vi "Advantech.vi"(8 "error in (no error)":errorcluster) -> (0 "error out":errorcluster, 3 "Advantech":T1)   [LabVIEW 2012]
panel:
  out "Array":dbl[](array[numeric])
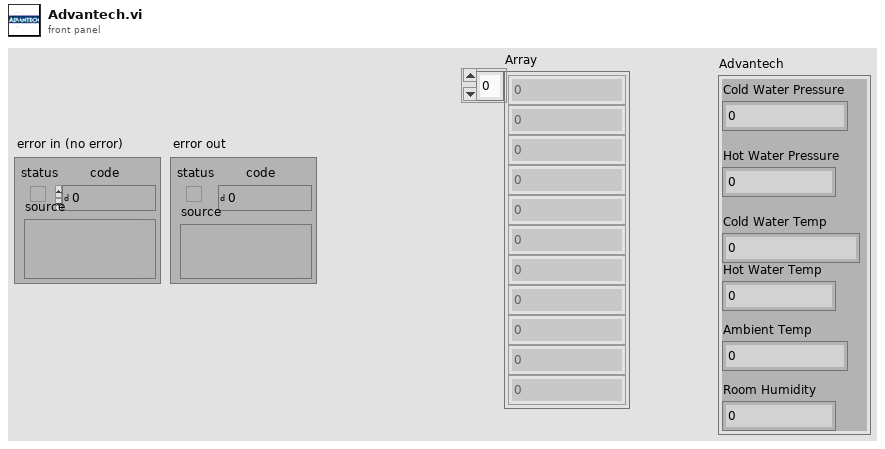
[diagram p1: front panel]
types:
  T1 = cluster{"Cold Water Pressure":dbl, "Hot Water Pressure":dbl, "Cold Water Temp":dbl, "Hot Water Temp":dbl, "Ambient Temp":dbl, "Room Humidity":dbl}
  T2 = cluster{"CP":dbl, "HP":dbl, "F1":dbl, "F2":dbl, "AT":dbl, "RH":dbl}
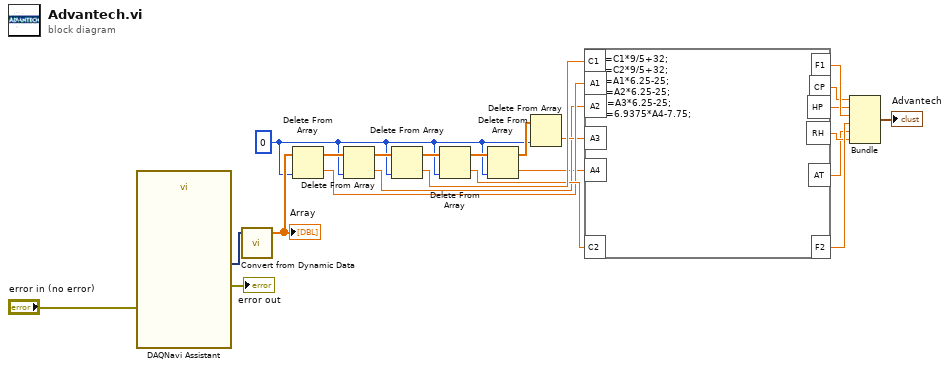
[diagram p0: block diagram]
diagram:
  w14 = 0 ("index")
  n1 = call "DAQNavi Assistant"("error in(no error)"="error in (no error)") -> ("error out"=→"error out":errorcluster, "data out(DDT)"=w21:dynamicdata)  [unwired: 17 in]
  n2 = call "Convert from Dynamic Data"("Dynamic Data Type"=w21) -> ("Array"=w20:dbl[])  [unwired: 3 in]
  "Array" <- w20
  n3 = Delete From Array(array=w20, index=w14) -> (deleted portion=w8:dbl, array with subset deleted=w19:dbl[])  [unwired: 1 in]
  n4 = Delete From Array(array=w19, index=w14) -> (deleted portion=w4:dbl, array with subset deleted=w18:dbl[])  [unwired: 1 in]
  n5 = Delete From Array(array=w18, index=w14) -> (deleted portion=w12:dbl, array with subset deleted=w17:dbl[])  [unwired: 1 in]
  n6 = Delete From Array(array=w17, index=w14) -> (deleted portion=w11:dbl, array with subset deleted=w16:dbl[])  [unwired: 1 in]
  n7 = Delete From Array(array=w16, index=w14) -> (deleted portion=w2:dbl, array with subset deleted=w15:dbl[])  [unwired: 1 in]
  n8 = Delete From Array(array=w15, index=w14) -> (deleted portion=w7:dbl)  [unwired: 1 in, 1 out]
  n9 = formula code="F1=C1*9/5+32;\nF2=C2*9/5+32;\nCP=A1*6.25-25;\nHP=A2*6.25-25;\nRH=A3*6.25-25;\nAT=6.9375*A4-7.75;"("C1"=w12, "C2"=w11, "A1"=w8, "A2"=w4, "A3"=w7, "A4"=w2) -> ("F1"=w10:dbl, "F2"=w9:dbl, "CP"=w5:dbl, "HP"=w3:dbl, "RH"=w6:dbl, "AT"=w1:dbl)
  n10 = Bundle("CP"=w5, "HP"=w3, "F1"=w10, "F2"=w9, "AT"=w1, "RH"=w6) -> (→"Advantech":T2)  [unwired: 1 in]
